vi "VLC - Save Audio Stream.vi"(5 "Media Source":string="rtsp://user:password@IPaddress/axis-media/media.amp?videocodec=h264", 7 "Script":string="sout=#transcode{acodec=mpga,ab=128,scale=1,channels=2,novideo}:duplicate{select=audio,dst=standard{access=file,dst='C:\\Audio\\Output.mp4'},dst=display{novideo}}", 11 "error in (no error)":errorcluster) -> (15 "error out":errorcluster)   [LabVIEW 2011]
panel:
  # "http://www.videolan.org/developers/vlc/doc/doxygen/html/modules.html"
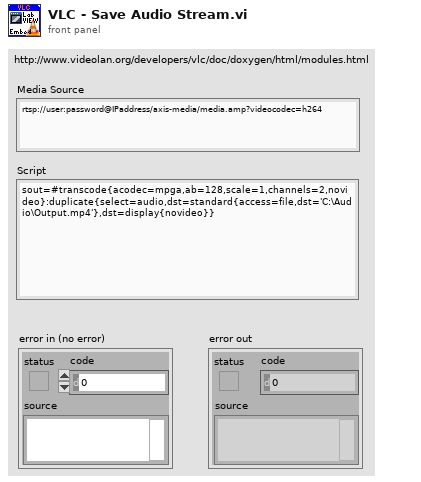
[diagram p1: front panel]
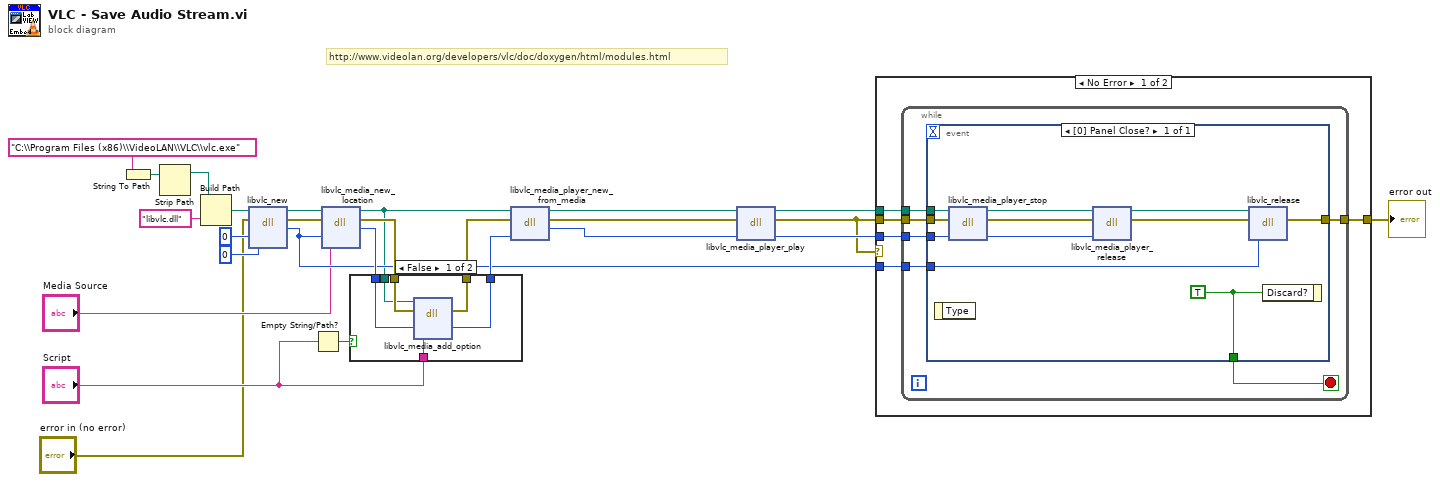
[diagram p0: block diagram]
diagram:
  # "http://www.videolan.org/developers/vlc/doc/doxygen/html/modules.html"
  n1 = String To Path(string="C:\\Program Files (x86)\\VideoLAN\\VLC\\vlc.exe") -> (path=w15:path)
  n2 = Strip Path(path=w15) -> (stripped path=w14:path)  [unwired: 1 out]
  n3 = Build Path(base path=w14, name or relative path="libvlc.dll") -> (appended path=w12:path)
  n4 = dll-call lib="C:/Program Files (x86)/VideoLAN/VLC/libvlc.dll" fn="libvlc_new"(path in=w12, error in="error in (no error)", "argc"=i16 0, "argv"=u8 0) -> (path out=w17:path, error out=w20:errorcluster, "return type"=w22:i32)  [unwired: 3 in]
  n5 = Empty String/Path?(string/path="Script") -> (empty?=w9:bool)
  n6 = dll-call lib="C:/Program Files (x86)/VideoLAN/VLC/libvlc.dll" fn="libvlc_media_new_location"(path in=w17, error in=w20, "p_instance"=w22, "path"="Media Source") -> (path out=w6:path, error out=w23:errorcluster, "return type"=w24:i32)  [unwired: 3 in]
  n7 = case shown="False" w9 {
    tunnel: w23 -> [w32 w34]
    tunnel: w24 -> [w31 w33]
    tunnel: [w30 w33] -> w25
    tunnel: [w29 w34] -> w26
    tunnel: "Script" -> [w28 _]
    tunnel: w6 -> [w27 _]
    frame False {
      n8 = dll-call lib="C:/Program Files (x86)/VideoLAN/VLC/libvlc.dll" fn="libvlc_media_add_option"(path in=w27, error in=w32, "p_md"=w31, "ppsz_options"=w28) -> (error out=w29:errorcluster, "p_md"=w30:i32)  [unwired: 3 in, 1 out]
    }
    frame True {
    }
  }
  n9 = dll-call lib="C:/Program Files (x86)/VideoLAN/VLC/libvlc.dll" fn="libvlc_media_player_new_from_media"(path in=w6, error in=w26, "p_md"=w25) -> (path out=w3:path, error out=w2:errorcluster, "return type"=w1:i32)  [unwired: 2 in]
  n10 = dll-call lib="C:/Program Files (x86)/VideoLAN/VLC/libvlc.dll" fn="libvlc_media_player_play"(path in=w3, error in=w2, "p_mi"=w1) -> (path out=w16:path, error out=w7:errorcluster, "p_mi"=w21:i32)  [unwired: 2 in]
  n11 = case shown="No Error" w7 {
    tunnel: w22 -> [w39 _]
    tunnel: w21 -> [w38 _]
    tunnel: w7 -> [w37 w57]
    tunnel: w16 -> [w36 _]
    tunnel: [w35 w57] -> w8
    frame No Error {
      n12 = while {
        tunnel: w39 -> [w45]
        tunnel: w38 -> [w44]
        tunnel: w37 -> [w43]
        tunnel: w36 -> [w42]
        tunnel: [w41] -> w35
        stop <- w40 stop-if-true
        n13 = event shown="[0] Panel Close?" {
          selector: _ -> [_]
          dyn-events: _ -> [_]
          timeout: _ -> [_]
          tunnel: w43 -> [w56]
          tunnel: w44 -> [w55]
          tunnel: w45 -> [w51]
          tunnel: w42 -> [w50]
          tunnel: [w47] -> w41
          tunnel: [w46] -> w40
          event Panel Close? {
            w46 = TRUE ("Discard?")
            n14 = event-data() -> ()  [unwired: 1 in, 1 out]
            n15 = dll-call lib="C:/Program Files (x86)/VideoLAN/VLC/libvlc.dll" fn="libvlc_media_player_stop"(path in=w50, error in=w56, "p_mi"=w55) -> (path out=w49:path, error out=w54:errorcluster, "p_mi"=w53:i32)  [unwired: 2 in]
            n16 = dll-call lib="C:/Program Files (x86)/VideoLAN/VLC/libvlc.dll" fn="libvlc_media_player_release"(path in=w49, error in=w54, "p_mi"=w53) -> (path out=w48:path, error out=w52:errorcluster)  [unwired: 3 in]
            n17 = dll-call lib="C:/Program Files (x86)/VideoLAN/VLC/libvlc.dll" fn="libvlc_release"(path in=w48, error in=w52, "p_instnace"=w51) -> (error out=w47:errorcluster)  [unwired: 3 in, 1 out]
            n18 = event-data("Discard?"=w46) -> ()  [unwired: 1 in, 1 out]
          }
        }
      }
    }
    frame Error {
    }
  }
  "error out" <- w8
